vi "target.vi"() -> ()   [LabVIEW 2020]
uses:
  <vilib>/rvi/interface/RandomDataEmulation/niFpgaRandomDataHandleErrors.vi
  <vilib>/rvi/DataTransferAndStorage/Container/XNode/niFpgaContainer.xnode
  <vilib>/rvi/interface/RandomDataEmulation/nirviRandomDataFpgaReadWriteTemplate.vi
panel:
  out "Timed Out? FIFO in REAL":bool
  out "Timed Out? FIFO out index":bool
  out "Timed Out? FIFO out REAL":bool
  out "sort time (us)":u32
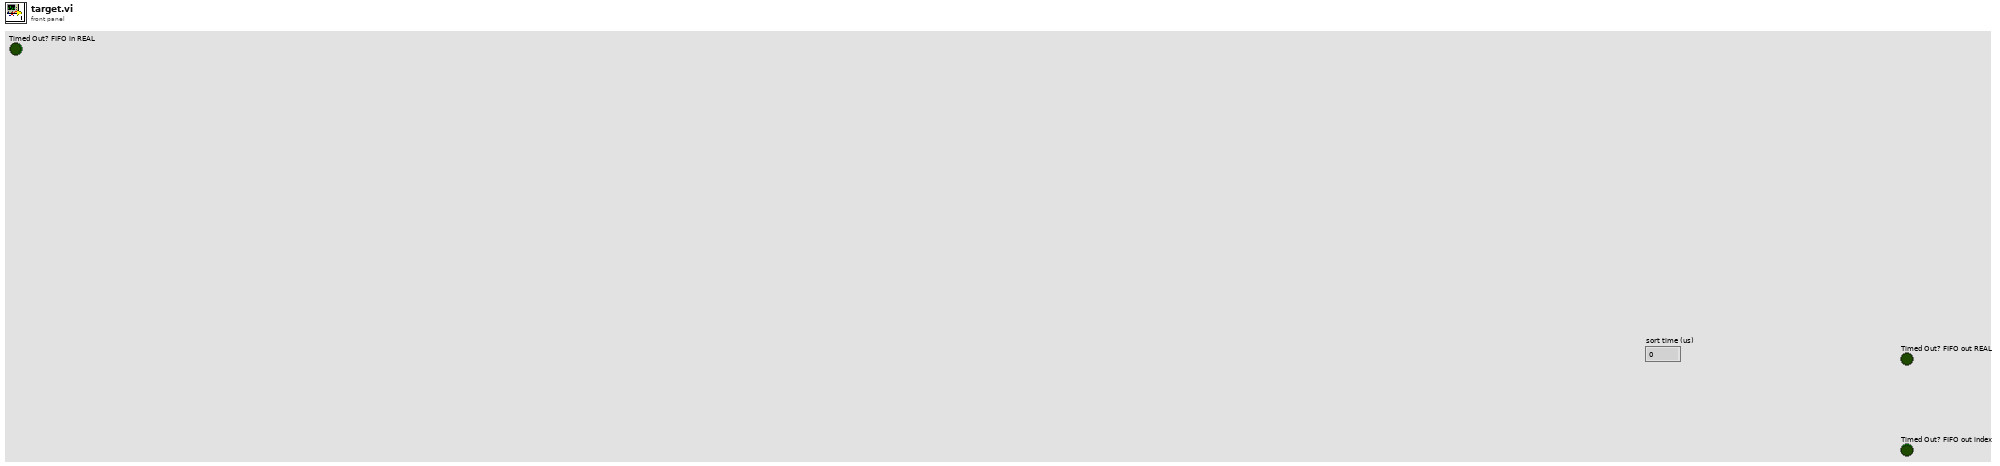
[diagram p1: front panel]
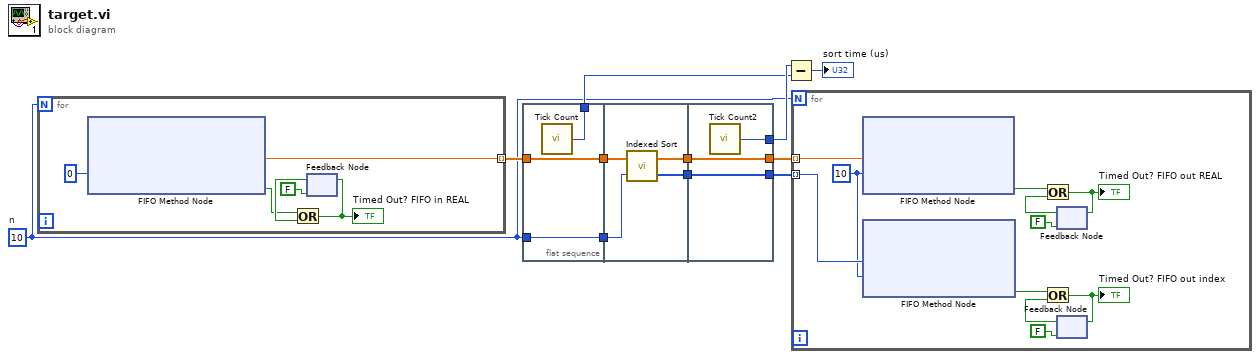
[diagram p0: block diagram]
diagram:
  w2 = 10  # n
  n1 = for {
    N: w2 -> [_]
    tunnel: [w12] -> w8 mode=indexing
    n2 = xnode ("FIFO Method Node")("Timeout"=0) -> ("Element"=w12:sgl, "Timed Out?"=w13:bool)  [unwired: 1 in, 1 out]
    n3 = feedback #1(FALSE) -> (w14:bool)
    n4 = Or(x=w13, y=w14) -> (x .or. y?=w15:bool)
    "Timed Out? FIFO in REAL" <- w15
    n5 = feedback-in #1(w15) -> ()
  }
  n6 = flat-sequence {
    tunnel: [w20] -> w10
    tunnel: w8 -> [w19]
    tunnel: [w19] -> w7
    tunnel: w2 -> [w18]
    tunnel: [w18] -> w1
    tunnel: w7 -> [w24]
    tunnel: [w22] -> w6
    tunnel: [w23] -> w3
    tunnel: w1 -> [w21]
    tunnel: [w27] -> w11
    tunnel: [w26] -> w5
    tunnel: w6 -> [w26]
    tunnel: [w25] -> w4
    tunnel: w3 -> [w25]
    frame #0 {
      n7 = call "Tick Count"() -> ("Tick Count(uSec)"=w20:u32)
    }
    frame #1 {
      n8 = call <vilib>:"Indexed Sort.vi"("n"=w21, "A"=w24) -> ("Index"=w23:i32[], "A Sorted"=w22:sgl[])
    }
    frame #2 {
      n9 = call "Tick Count2"() -> ("Tick Count(uSec)"=w27:u32)
    }
  }
  n10 = Subtract(x=w11, y=w10) -> (x-y=→"sort time (us)":u32)
  n11 = for {
    N: w2 -> [_]
    tunnel: w4 -> [w38] mode=indexing
    tunnel: w5 -> [w37] mode=indexing
    w36 = 10 ("Timeout")
    n12 = xnode ("FIFO Method Node")("Element"=w37, "Timeout"=w36) -> ("Timed Out?"=w32:bool)  [unwired: 1 in, 1 out]
    n13 = xnode ("FIFO Method Node")("Element"=w38, "Timeout"=w36) -> ("Timed Out?"=w28:bool)  [unwired: 1 in, 1 out]
    n14 = feedback #2(FALSE) -> (w33:bool)
    n15 = Or(x=w32, y=w33) -> (x .or. y?=w34:bool)
    "Timed Out? FIFO out REAL" <- w34
    n16 = feedback-in #2(w34) -> ()
    n17 = feedback #3(FALSE) -> (w31:bool)
    n18 = Or(x=w28, y=w31) -> (x .or. y?=w30:bool)
    "Timed Out? FIFO out index" <- w30
    n19 = feedback-in #3(w30) -> ()
  }
